vi "Clippy_Create.vi"(8 "error in (no error)":errorcluster, 9 "AnswerRef":refnum<vi>, 10 "ClippyPictureRef":refnum<vi>, 11 "reference in":refnum<class "Clippy.lvclass">) -> (0 "error out":errorcluster, 3 "reference out":refnum<class "Clippy.lvclass">)   [LabVIEW 2020, in "Clippy.lvclass"]
uses:
  Clippy.lvclass
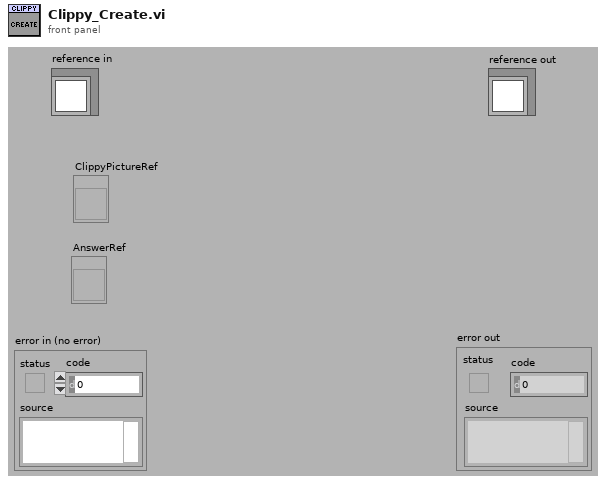
[diagram p1: front panel]
types:
  T1 = typedef "Clippy.lvclass/ObjectAttributes.ctl" = cluster{"ClippyPictureRef":refnum<vi>, "LastAnimation":T2, "LastAnimated":timestamp, "Visible":bool, "AnswerRef":refnum<vi>}
  T2 = typedef "Clippy.lvclass/AnimationTypes.ctl" = enum16{"Congratulate", "LookRight", "SendMail", "Thinking", "Explain", "IdleRopePile", "IdleAtom", "Print", "Hide", "GetAttention", "Save", "GetTechy", "GestureUp", "Idle1_1", "Processing", "Alert", "LookUpRight", "IdleSideToSide", "GoodBye", "LookLeft", "IdleHeadScratch", "LookUpLeft", "CheckingSomething", "Hearing_1", "GetWizardy", "IdleFingerTap", "GestureLeft", "Wave", "GestureRight", "Writing", "IdleSnooze", "LookDownRight", "GetArtsy", "Show", "LookDown", "Searching", "EmptyTrash", "Greeting", "LookUp", "GestureDown", "RestPose", "IdleEyeBrowRaise", "LookDownLeft"}
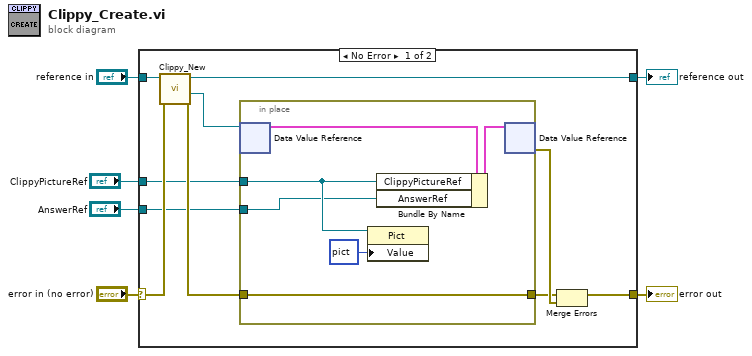
[diagram p0: block diagram]
diagram:
  n1 = case shown="No Error" "error in (no error)" {
    selector: "error in (no error)" -> [w15 w24]
    tunnel: [w9 w24] -> w5
    tunnel: "reference in" -> [w16 w23]
    tunnel: [w14 w23] -> w3
    tunnel: "ClippyPictureRef" -> [w8 _]
    tunnel: "AnswerRef" -> [w7 _]
    frame No Error {
      n2 = call "Clippy_New.vi"("error in (no error)"=w15, "reference in"=w16) -> ("error out"=w11:errorcluster, "DVRRefOut"=w12:refnum<data-value>, "reference out"=w14:refnum<class "Clippy.lvclass">)  [unwired: 6 in, 1 out]
      n3 = in-place {
        in-place-border: w11 -> [w20]
        in-place-border: [w20] -> w10
        in-place-border: w8 -> [w19]
        in-place-border: w7 -> [w17]
        n4 = in-place-dvr #1(w12) -> (w21:T1)  [unwired: 1 out]
        n5 = property class="Pict"(reference=w19, "Value"=picture data[5B]) -> ()  [unwired: 1 in, 2 out]
        n6 = Bundle By Name(cluster=w21, "ClippyPictureRef"=w19, "AnswerRef"=w17) -> (w22:T1)
        n7 = in-place-dvr #1(w22) -> (w13:errorcluster)  [unwired: 1 out]
      }
      n8 = Merge Errors(w10, w13) -> (w9:errorcluster)
    }
    frame Error {
      # "VI-TechBaseTemplate_Simple_4x4x4"
    }
  }
  "error out" <- w5
  "reference out" <- w3
